vi "Enable All Axes.vi"(8 "error in (no error)":errorcluster, 11 "Gantry In":refnum<k24>) -> (0 "error out":errorcluster, 3 "Gantry Out":refnum<k24>)   [LabVIEW 2018, in "A3200.lvclass"]
uses:
  A3200.lvclass
  C:/Program Files (x86)/Aerotech/A3200/LabVIEW/2010/Bin/Aerotech.A3200.dll
  Program Files (x86)/Aerotech/A3200/LabVIEW/2010/Bin/Aerotech.A3200.dll
  Drivers/Aerotech A3200/Aerotech.lvlib
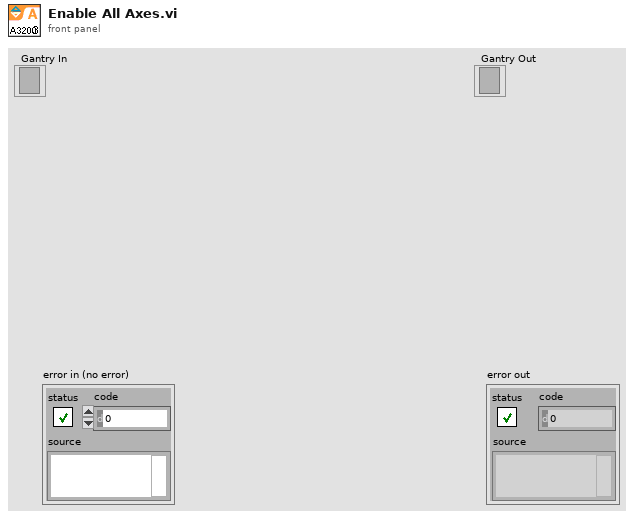
[diagram p1: front panel]
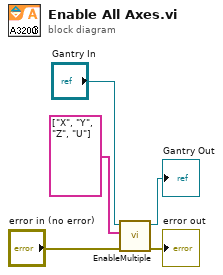
[diagram p0: block diagram]
diagram:
  n1 = call "EnableMultiple.vi"("error in (no error)"="error in (no error)", "axis names"=string[] ["X", "Y", "Z", "U"], "controller in"="Gantry In") -> ("error out"=→"error out":errorcluster, "controller out"=→"Gantry Out":refnum<k24>)  [unwired: 7 in]
